vi "g.vi"(6 "Variant in":variant, 7 "Shift Pressed?":bool, 8 "error in (no error)":errorcluster, 10 "QD Combo Box Ref":refnum<vi>, 11 "QD Launch VI Ref":refnum<vi>) -> (0 "error out":errorcluster, 4 "Variant out":variant)   [LabVIEW 2009]
panel:
  # "Do not change the connector pane of this VI."
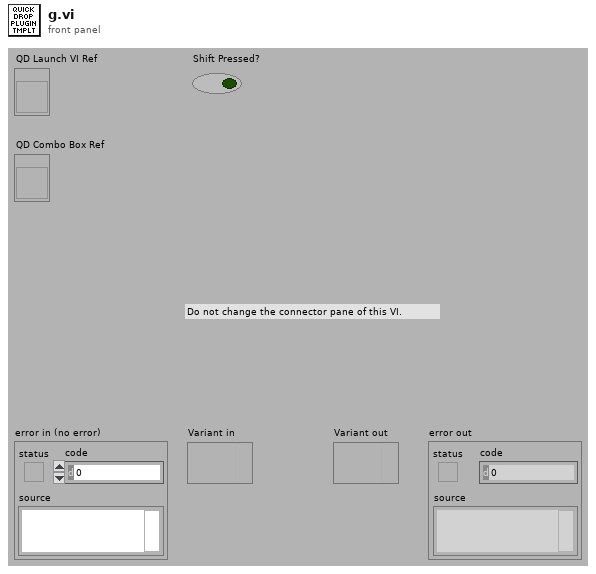
[diagram p1: front panel]
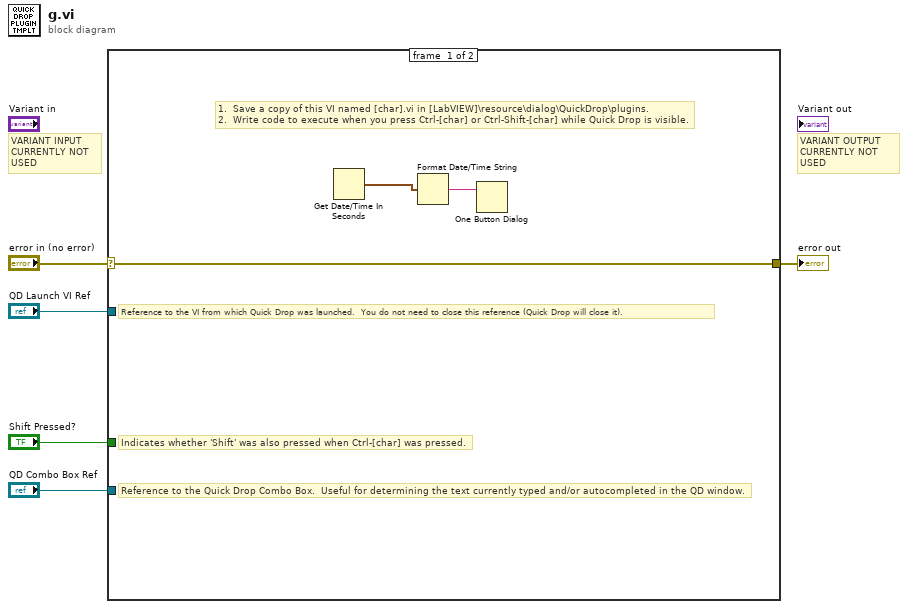
[diagram p0: block diagram]
diagram:
  # "VARIANT INPUT\nCURRENTLY NOT\nUSED"
  # "VARIANT OUTPUT\nCURRENTLY NOT\nUSED"
  n1 = case shown="Pas d'erreur" "error in (no error)" {
    selector: "error in (no error)" -> [w8 w9]
    tunnel: [w8 w9] -> w4
    tunnel: "QD Launch VI Ref" -> [_ _]
    tunnel: "Shift Pressed?" -> [_ _]
    tunnel: "QD Combo Box Ref" -> [_ _]
    frame #0 {
      # "Reference to the VI from which Quick Drop was launched.  You do not need to close this reference (Quick Drop will close it)."
      # "Reference to the Quick Drop Combo Box.  Useful for determining the text currently typed and/or autocompleted in the QD window."
      # "Indicates whether 'Shift' was also pressed when Ctrl-[char] was pressed."
      # "1.  Save a copy of this VI named [char].vi in [LabVIEW]\\resource\\dialog\\QuickDrop\\plugins.\n2.  Write code to execute when you press Ctrl-[char] or Ctrl-Shift-[char] while Quick Drop is visible."
      n2 = Get Date/Time In Seconds() -> (seconds since 1Jan1904=w7:timestamp)
      n3 = Format Date/Time String(seconds (now)=w7) -> (date/time string=w6:string)  [unwired: 2 in]
      n4 = One Button Dialog(message=w6) -> ()  [unwired: 1 in, 1 out]
    }
    frame #1 {
    }
  }
  "error out" <- w4
